vi "eFGV - Page Name List.vi"(6 "Action":T1, 8 "Error In":errorcluster, 11 "Enable Page In":string[](array[string])) -> (0 "Error Out":errorcluster, 2 "Event Enable Page":refnum<user-event>, 3 "Enable Page Out":string[](array[string]))   [LabVIEW 2020]
uses:
  Control/State - eFGV.ctl
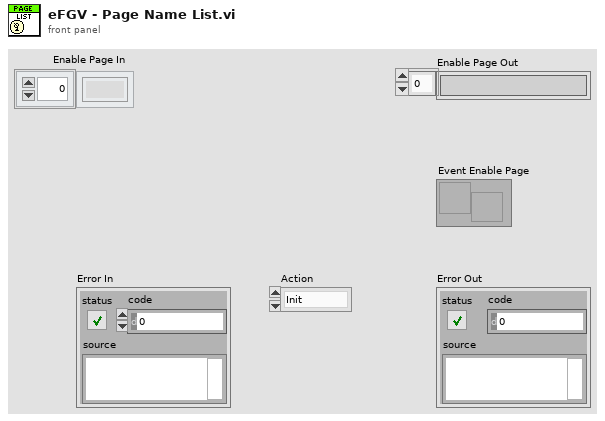
[diagram p1: front panel]
types:
  T1 = typedef "State - eFGV.ctl" = enum16{"Init", "Read", "Write", "Exit"}
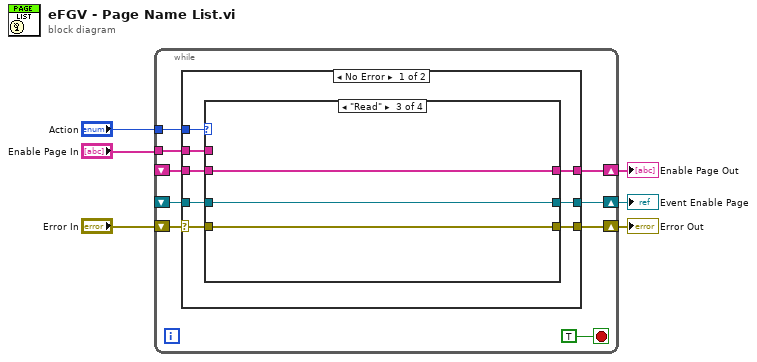
[diagram p0: block diagram]
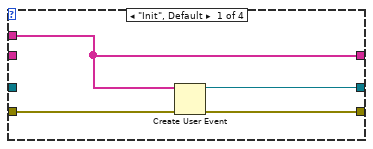
[diagram p2: hidden frame]
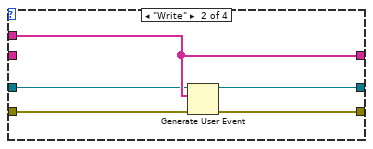
[diagram p3: hidden frame]
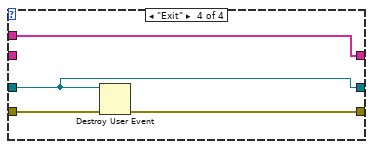
[diagram p4: hidden frame]
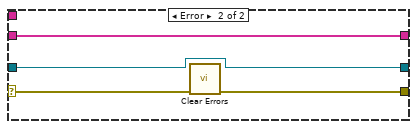
[diagram p5: hidden frame]
diagram:
  n1 = while {
    shift-right: [w14] -> w5
    shift-left: "Error In" -> [w15]
    tunnel: "Action" -> [w13]
    tunnel: "Enable Page In" -> [w11]
    shift-right: [w10] -> w2
    shift-left: _ -> [w9]
    shift-right: [w7] -> w1
    shift-left: _ -> [w8]
    stop <- TRUE stop-if-true
    n2 = case shown="No Error" w15 {
      selector: w15 -> [w23 w43]
      tunnel: w13 -> [w21 _]
      tunnel: [w22 w42] -> w14
      tunnel: w11 -> [w20 _]
      tunnel: [w19 w41] -> w10
      tunnel: w9 -> [w18 w41]
      tunnel: w8 -> [w17 w40]
      tunnel: [w16 w40] -> w7
      frame No Error {
        n3 = case shown="\"Read\"" w21 {
          tunnel: w23 -> [w27 w32 w35 w39]
          tunnel: [w26 w31 w35 w38] -> w22
          tunnel: w20 -> [w25 w30 _ w37]
          tunnel: [w25 w30 w34 w37] -> w19
          tunnel: w18 -> [_ _ w34 _]
          tunnel: w17 -> [_ w28 w33 w36]
          tunnel: [w24 w29 w33 w36] -> w16
          frame "Init", Default {
            n4 = Create User Event(user event datatype=w25, error in=w27) -> (user event=w24:refnum<user-event>, error out=w26:errorcluster)
          }
          frame "Write" {
            n5 = Generate User Event(user event=w28, event data cluster=w30, error in=w32) -> (user event out=w29:refnum<user-event>, error out=w31:errorcluster)  [unwired: 1 in]
          }
          frame "Read" {
          }
          frame "Exit" {
            n6 = Destroy User Event(user event=w36, error in=w39) -> (error out=w38:errorcluster)
          }
        }
      }
      frame Error {
        n7 = call <vilib>:"Clear Errors.vi"("error in (no error)"=w43) -> ("error out"=w42:errorcluster)  [unwired: 5 in, 1 out]
      }
    }
  }
  "Error Out" <- w5
  "Enable Page Out" <- w2
  "Event Enable Page" <- w1
